vi "EnumControls-OutOfRange.vi"(0 "Test Case":T5(ring), 5 "Enum":enum16{"Zero", "One", "Two", "Three"}(ring)=enum."Three", 7 "Array Of Enums":enum16{"Cero", "Uno", "Dos", "Tres"}[](array[ring])=[enum."Dos", enum."Uno", enum."Dos"], 9 "Cluster":T3={"Enum In Cluster (U8)"=enum."One", "Enum 2 In Cluster"=enum."Two", "Array In Cluster (U32)"=[enum."Zero", enum."One", enum."Two"]}, 11 "Array Of Clusters":T4(array[cluster])=[{"Numbers In Spanish"=enum."Uno", "Array"=[enum."Uno", enum."Dos", enum."Uno"]}, {"Numbers In Spanish"=enum."Cero", "Array"=[enum."Cero", enum."Cero", enum."Cero"]}, {"Numbers In Spanish"=enum."Dos", "Array"=[enum."Dos", enum."Dos", enum."Dos"]}]) -> (2 "Enum Out":enum16{"Zero", "One", "Two", "Three"}(ring)=enum."Three", 3 "Array Of Enums Out":enum16{"Cero", "Uno", "Dos", "Tres"}[](array[ring])=[enum."Dos", enum."Uno", enum."Dos"], 4 "Cluster Out":T3={"Enum In Cluster (U8)"=enum."One", "Enum 2 In Cluster"=enum."Two", "Array In Cluster (U32)"=[enum."Zero", enum."One", enum."Two"]}, 6 "Array Of Clusters Out":T4(array[cluster])=[{"Numbers In Spanish"=enum."Uno", "Array"=[enum."Uno", enum."Dos", enum."Uno"]}, {"Numbers In Spanish"=enum."Cero", "Array"=[enum."Cero", enum."Cero", enum."Cero"]}, {"Numbers In Spanish"=enum."Dos", "Array"=[enum."Dos", enum."Dos", enum."Dos"]}], 8 "Numeric Out":i16=-25, 10 "Array Of Numbers Out":i16[](array[numeric])=[-45, 12345, 3], 13 "Got Expected Values":bool, 14 "Array Of Clusters (Numeric) Out":T2(array[cluster])=[{"Numbers In Spanish"=-12, "Array"=[-45, 1234]}, {"Numbers In Spanish"=1, "Array"=[-3, -2, 111]}, {"Numbers In Spanish"=3, "Array"=[]}], 15 "Cluster (Numeric) Out":T1={"Enum In Cluster (U8)"=-120, "Enum 2 In Cluster"=789, "Array In Cluster (U32)"=[1234567, 1, 3, -45789]})   [LabVIEW 2012]
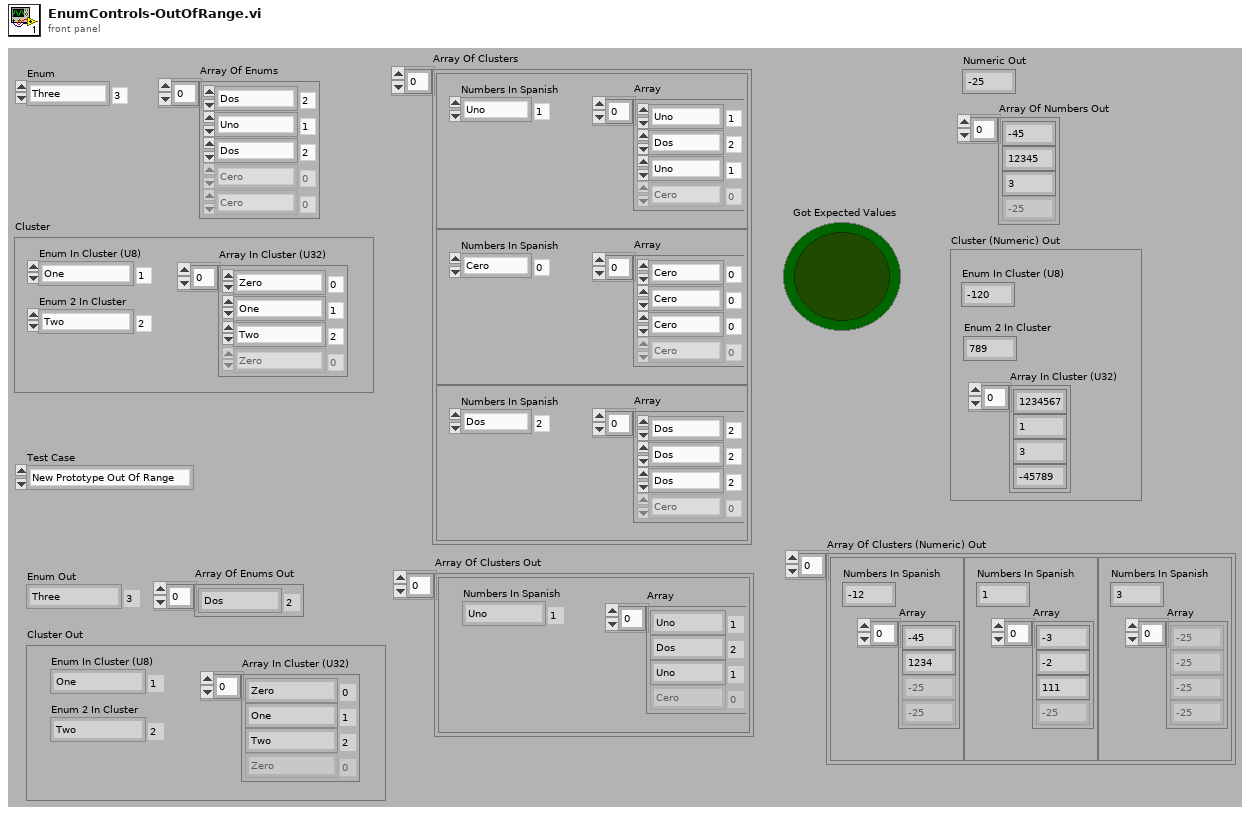
[diagram p1: front panel]
types:
  T1 = cluster{"Enum In Cluster (U8)":i8, "Enum 2 In Cluster":i16, "Array In Cluster (U32)":i32[]}
  T2 = cluster{"Numbers In Spanish":i16, "Array":i16[]}[]
  T3 = cluster{"Enum In Cluster (U8)":enum8{"Zero", "One", "Two", "Three"}, "Enum 2 In Cluster":enum16{"Zero", "One", "Two", "Three"}, "Array In Cluster (U32)":enum32{"Zero", "One", "Two", "Three"}[]}
  T4 = cluster{"Numbers In Spanish":enum16{"Cero", "Uno", "Dos", "Tres"}, "Array":enum16{"Cero", "Uno", "Dos", "Tres"}[]}[]
  T5 = enum16{"New Prototype Out Of Range", "Old Prototype Out Of Range"}
  T6 = cluster{"Enum In Cluster":enum8{"Zero", "One", "Two", "Three"}, "Enum 2 In Cluster":enum16{"Zero", "One", "Two", "Three"}, "Array In Cluster":enum32{"Zero", "One", "Two", "Three"}[]}
  T7 = cluster{"Numbers In Spanish":bool, "Array":bool[]}[]
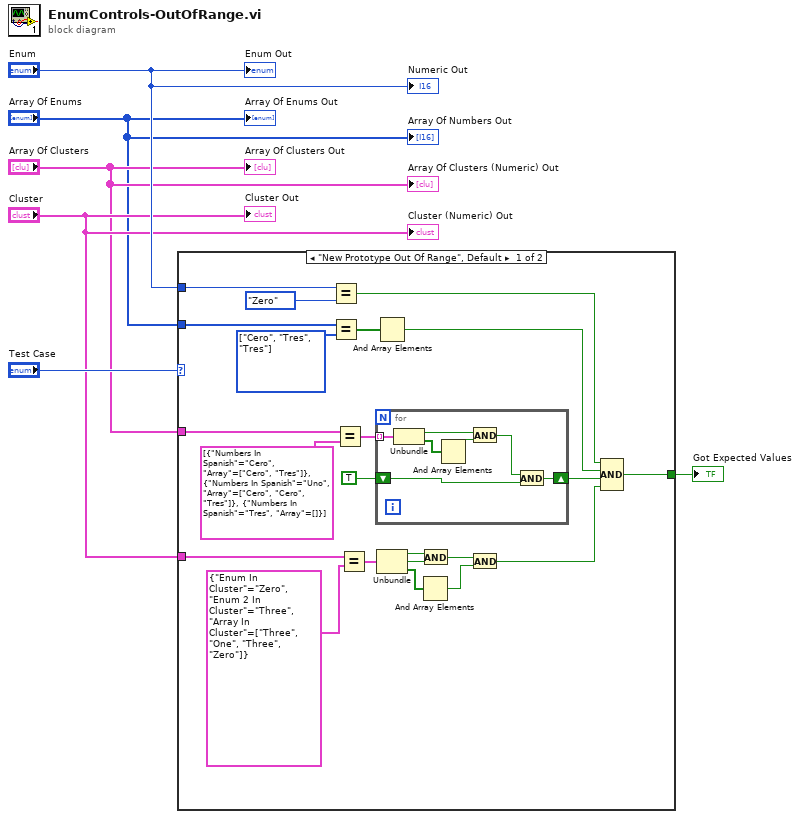
[diagram p0: block diagram]
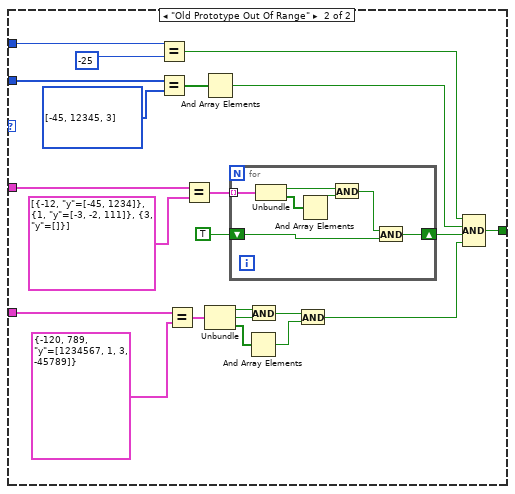
[diagram p2: hidden frame]
diagram:
  n1 = case shown="\"New Prototype Out Of Range\", Default" "Test Case" {
    tunnel: "Enum" -> [w9 w41]
    tunnel: "Array Of Enums" -> [w7 w40]
    tunnel: "Array Of Clusters" -> [w11 w39]
    tunnel: "Cluster" -> [w10 w38]
    tunnel: [w8 w36] -> w5
    frame "New Prototype Out Of Range", Default {
      w27 = enum16{"Cero", "Uno", "Dos", "Tres"}[] [enum."Cero", enum."Tres", enum."Tres"] items=["Cero", "Uno", "Dos", "Tres"] ("y")
      n2 = Equal?(x=w9, y=enum16{"Zero", "One", "Two", "Three"}."Zero") -> (x = y?=w19:bool)
      n3 = Equal?(x=w7, y=w27) -> (x = y?=w24:bool[])
      n4 = Equal?(x=w11, y=T4 [{"Numbers In Spanish"=enum."Cero", "Array"=[enum."Cero", enum."Tres"]}, {"Numbers In Spanish"=enum."Uno", "Array"=[enum."Cero", enum."Cero", enum."Tres"]}, {"Numbers In Spanish"=enum."Tres", "Array"=[]}]) -> (x = y?=w14:T7)
      n5 = Equal?(x=w10, y=T6 {"Enum In Cluster"=enum."Zero", "Enum 2 In Cluster"=enum."Three", "Array In Cluster"=[enum."Three", enum."One", enum."Three", enum."Zero"]}) -> (x = y?=w23:cluster{bool, "Enum 2 In Cluster":bool, bool[]})
      n6 = for {
        tunnel: w14 -> [w35] mode=indexing
        shift-right: [w29] -> w12
        shift-left: TRUE -> [w30]
        n7 = Unbundle(w35) -> ("Numbers In Spanish"=w33:bool, "Array"=w34:bool[])
        n8 = And Array Elements(Boolean array=w34) -> (logical AND=w32:bool)
        n9 = And(x=w33, y=w32) -> (x .and. y?=w31:bool)
        n10 = And(x=w31, y=w30) -> (x .and. y?=w29:bool)
      }
      n11 = And Array Elements(Boolean array=w24) -> (logical AND=w18:bool)
      n12 = Unbundle(w23) -> (w21:bool, "Enum 2 In Cluster"=w20:bool, w22:bool[])
      n13 = And Array Elements(Boolean array=w22) -> (logical AND=w17:bool)
      n14 = And(x=w21, y=w20) -> (x .and. y?=w16:bool)
      n15 = And(x=w16, y=w17) -> (x .and. y?=w15:bool)
      n16 = Compound Arithmetic op=AND(w19, w18, w12, w15) -> (w8:bool)
    }
    frame "Old Prototype Out Of Range" {
      n17 = Equal?(x=w41, y=i16 -25) -> (x = y?=w49:bool)
      n18 = Equal?(x=w40, y=i16[] [-45, 12345, 3]) -> (x = y?=w54:bool[])
      n19 = Equal?(x=w38, y=cluster{i8, i16, "y":i32[]} {-120, 789, "y"=[1234567, 1, 3, -45789]}) -> (x = y?=w53:cluster{bool, bool, bool[]})
      n20 = Equal?(x=w39, y=cluster{i16, "y":i16[]}[] [{-12, "y"=[-45, 1234]}, {1, "y"=[-3, -2, 111]}, {3, "y"=[]}]) -> (x = y?=w44:cluster{bool, bool[]}[])
      n21 = And Array Elements(Boolean array=w54) -> (logical AND=w48:bool)
      n22 = Unbundle(w53) -> (w51:bool, w50:bool, w52:bool[])
      n23 = for {
        tunnel: w44 -> [w64] mode=indexing
        shift-right: [w58] -> w42
        shift-left: TRUE -> [w59]
        n24 = Unbundle(w64) -> (w62:bool, w63:bool[])
        n25 = And Array Elements(Boolean array=w63) -> (logical AND=w61:bool)
        n26 = And(x=w62, y=w61) -> (x .and. y?=w60:bool)
        n27 = And(x=w60, y=w59) -> (x .and. y?=w58:bool)
      }
      n28 = And Array Elements(Boolean array=w52) -> (logical AND=w47:bool)
      n29 = And(x=w51, y=w50) -> (x .and. y?=w46:bool)
      n30 = And(x=w46, y=w47) -> (x .and. y?=w45:bool)
      n31 = Compound Arithmetic op=AND(w49, w48, w42, w45) -> (w36:bool)
    }
  }
  "Got Expected Values" <- w5
  "Enum Out" <- "Enum"
  "Array Of Enums Out" <- "Array Of Enums"
  "Array Of Clusters Out" <- "Array Of Clusters"
  "Cluster Out" <- "Cluster"
  "Numeric Out" <- "Enum"
  "Array Of Numbers Out" <- "Array Of Enums"
  "Array Of Clusters (Numeric) Out" <- "Array Of Clusters"
  "Cluster (Numeric) Out" <- "Cluster"
